vi "Configure Measurement (Adjacent Channel Power).vi"(0 "VISA resource name":refnum<visa-resource-name>, 1 "Enable Limit Test (Enable)":bool, 2 "Method (0: Integration Bandwidth)":u16(ring) items=["Integration Bandwidth", "Resolution Bandwidth", "FAST"], 5 "Channel Integration Bandwidth (2E+6 Hz)":dbl=2000000.0 format="%#.6g", 7 "Measurement Type (0: Total Power Reference)":u16(ring) items=["Total Power Reference", "Power Spectral Density"], 9 "Enable Auto Reference (T: Enable)":bool=TRUE, 11 "error in (no error)":errorcluster, 12 "Manual Reference (10 dBm)":dbl=10.0 format="%#.6g") -> (4 "VISA resource name out":refnum<visa-resource-name>, 15 "error out":errorcluster)   [LabVIEW 2014, in "Agilent ESA PSA Series.lvlib"]
doc: "Sets up the adjacent channel power measurement operation."
uses:
  Agilent ESA PSA Series.lvlib
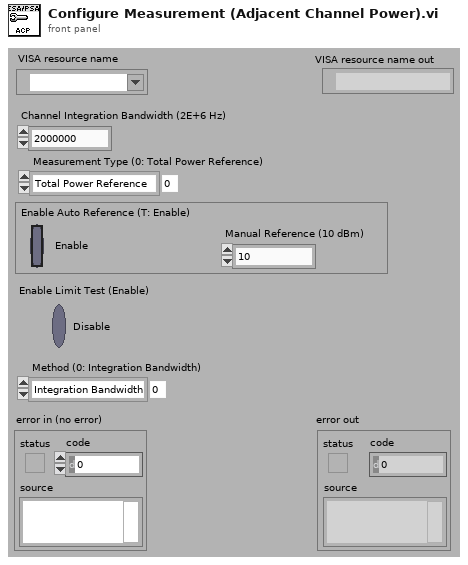
[diagram p1: front panel]
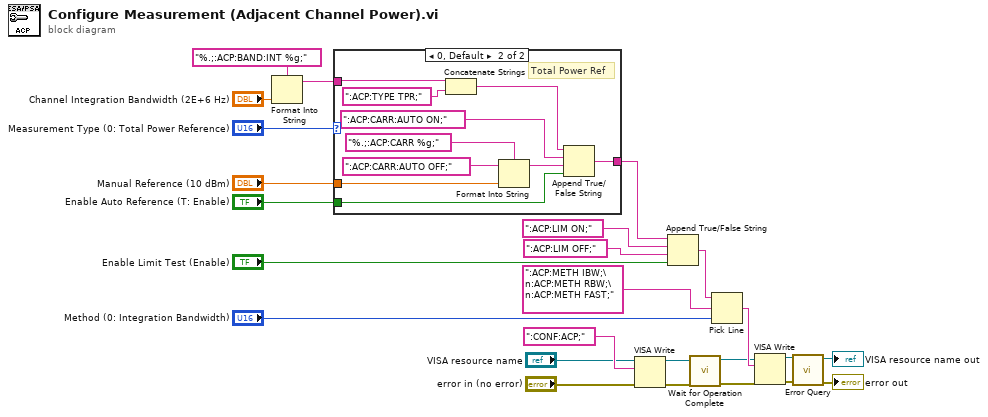
[diagram p0: block diagram]
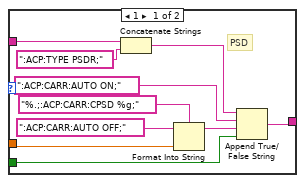
[diagram p2: hidden frame]
diagram:
  n1 = Format Into String(format string="%.;:ACP:BAND:INT %g;", "Channel Integration Bandwidth (2E+6 Hz)") -> (resulting string=w18:string)  [unwired: 2 in, 1 out]
  n2 = case shown="0, Default" "Measurement Type (0: Total Power Reference)" {
    tunnel: "Manual Reference (10 dBm)" -> [w31 w41]
    tunnel: "Enable Auto Reference (T: Enable)" -> [w30 w40]
    tunnel: w18 -> [w29 w38]
    tunnel: [w26 w36] -> w10
    frame 1 {
      # "PSD"
      n3 = Concatenate Strings(w29, ":ACP:TYPE PSDR;" ("string")) -> (w27:string)
      n4 = Format Into String(format string="%.;:ACP:CARR:CPSD %g;", initial string=":ACP:CARR:AUTO OFF;" ("true string"), w31) -> (resulting string=w34:string)  [unwired: 1 in, 1 out]
      n5 = Append True/False String(1:w30, 2:w34, 3:":ACP:CARR:AUTO ON;" ("true string"), 4:w27) -> (0:w26:string)
    }
    frame 0, Default {
      # "Total Power Ref"
      n6 = Concatenate Strings(w38, ":ACP:TYPE TPR;" ("string")) -> (w37:string)
      n7 = Format Into String(format string="%.;:ACP:CARR %g;", initial string=":ACP:CARR:AUTO OFF;" ("true string"), w41) -> (resulting string=w44:string)  [unwired: 1 in, 1 out]
      n8 = Append True/False String(1:w40, 2:w44, 3:":ACP:CARR:AUTO ON;" ("true string"), 4:w37) -> (0:w36:string)
    }
  }
  n9 = VISA Write(VISA resource name="VISA resource name", write buffer=":CONF:ACP;" ("initial string"), error in (no error)="error in (no error)") -> (VISA resource name out=w6:refnum<visa-resource-name>, error out=w5:errorcluster)  [unwired: 1 out]
  n10 = Append True/False String(1:"Enable Limit Test (Enable)", 2:":ACP:LIM OFF;" ("true string"), 3:":ACP:LIM ON;" ("true string"), 4:w10) -> (0:w12:string)
  n11 = call "Wait for Operation Complete.vi"("error in (no error)"=w5, "VISA resource name"=w6) -> ("error out"=w3:errorcluster, "VISA resource name out"=w4:refnum<visa-resource-name>)  [unwired: 8 in]
  n12 = Pick Line(string ("")=w12, multi-line string=":ACP:METH IBW;\n:ACP:METH RBW;\n:ACP:METH FAST;" ("format string"), line index="Method (0: Integration Bandwidth)") -> (output string=w11:string)
  n13 = VISA Write(VISA resource name=w4, write buffer=w11, error in (no error)=w3) -> (VISA resource name out=w2:refnum<visa-resource-name>, error out=w1:errorcluster)  [unwired: 1 out]
  n14 = call "Error Query.vi"("error in (no error)"=w1, "VISA resource name"=w2) -> ("error out"=→"error out":errorcluster, "VISA resource name out"=→"VISA resource name out":refnum<visa-resource-name>)  [unwired: 6 in, 2 out]
